vi "retrieveMonoSettings.vi"(8 "error in (no error)":errorcluster, 11 "ConfigurationFileReader in":refnum<class "ConfigurationFileReader.lvclass">) -> (0 "error out":errorcluster, 2 "Mono Settings":T1, 3 "ConfigurationFileReader out":refnum<class "ConfigurationFileReader.lvclass">)   [LabVIEW 2016, in "Settings.lvlib" / "ConfigurationFileReader.lvclass"]
uses:
  ConfigurationFileReader.lvclass
  ConfigurationTypedefs/Base/MonochromatorSettings.ctl
  Typedefs/wavelength.ctl
  Typedefs/slitWidth.ctl
  ConfigurationTypedefs/ConfigurationTypedefs.lvlib
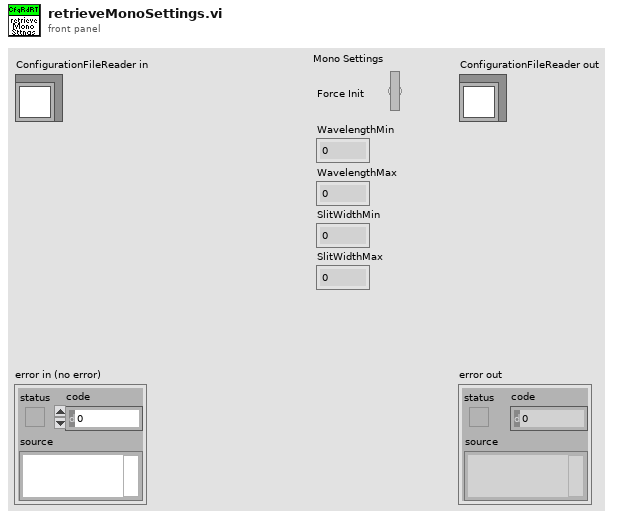
[diagram p1: front panel]
types:
  T1 = typedef "Settings.lvlib/ConfigurationTypedefs.lvlib/MonochromatorSettings.ctl" = cluster{"Force Init":bool, "WavelengthMin":T2, "WavelengthMax":T2, "SlitWidthMin":T3, "SlitWidthMax":T3}
  T2 = typedef "wavelength.ctl" = dbl
  T3 = typedef "slitWidth.ctl" = dbl
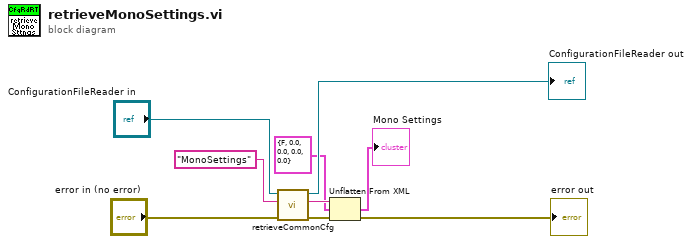
[diagram p0: block diagram]
diagram:
  n1 = call "retrieveCommonCfg.vi"("error in (no error)"="error in (no error)", "dataName"="MonoSettings", "ConfigurationFileReader in"="ConfigurationFileReader in") -> ("error out"=w4:errorcluster, "dataValueFromFile"=w5:string, "ConfigurationFileReader out"=→"ConfigurationFileReader out":refnum<class "ConfigurationFileReader.lvclass">)  [unwired: 6 in]
  n2 = Unflatten From XML(xml string=w5, type=T1 {"Force Init"=FALSE, "WavelengthMin"=0.0, "WavelengthMax"=0.0, "SlitWidthMin"=0.0, "SlitWidthMax"=0.0} ("SetLimits"), error in (no error)=w4) -> (value=→"Mono Settings":T1, error out=→"error out":errorcluster)
